vi "FreqC.Send Message.vi"(8 "error in":errorcluster, 9 "data":dbl, 10 "Message type":T1, 11 "FreqC Message queue in":refnum<queue>) -> (0 "error out":errorcluster, 3 "FreqC Message queue out":refnum<queue>)   [LabVIEW 2018]
uses:
  typedefs/FreqC.Message.ctl
  typedefs/FreqC.Message Type.ctl
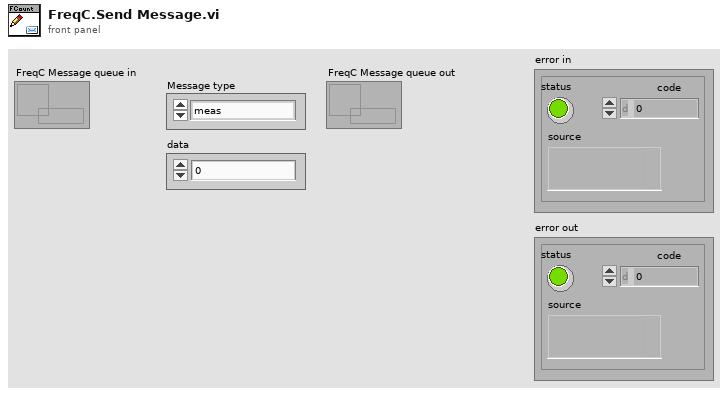
[diagram p1: front panel]
types:
  T1 = typedef "FreqC.Message Type.ctl" = enum16{"meas", "set level", "set gate"}
  T2 = typedef "FreqC.Message.ctl" = cluster{"Message type":T1, "data":dbl}
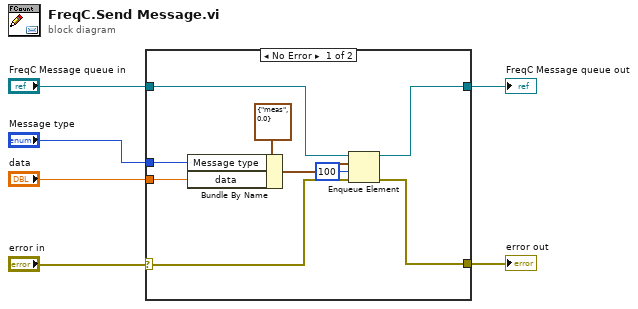
[diagram p0: block diagram]
diagram:
  n1 = case shown="No Error" "error in" {
    selector: "error in" -> [w10 w16]
    tunnel: "FreqC Message queue in" -> [w15 w17]
    tunnel: "Message type" -> [w13 _]
    tunnel: "data" -> [w11 _]
    tunnel: [w8 w16] -> w2
    tunnel: [w7 w17] -> w1
    frame No Error {
      n2 = Bundle By Name(cluster=T2 {"Message type"=enum."meas", "data"=0.0} ("element"), "Message type"=w13, "data"=w11) -> (w12:T2)
      n3 = Enqueue Element(queue=w15, element=w12, timeout in ms (-1)=100, error in (no error)=w10) -> (queue out=w7:refnum<queue>, error out=w8:errorcluster)  [unwired: 1 out]
    }
    frame Error {
    }
  }
  "error out" <- w2
  "FreqC Message queue out" <- w1
